vi "Assert ExcelReader Core.vi"() -> ()   [LabVIEW 2015, in "Admin_Actor.lvlib" / "ExcelReader.lvclass"]
uses:
  ExcelReader.lvclass
panel:
  in  "Path":path
  in  "ExcelReader in":refnum<class "ExcelReader.lvclass">
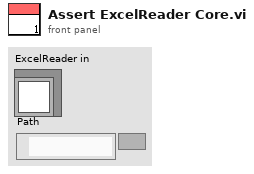
[diagram p1: front panel]
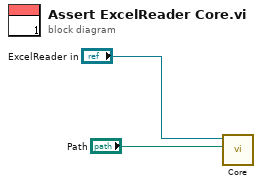
[diagram p0: block diagram]
diagram:
  n1 = call "Core.vi"("Path"="Path", "ExcelReader in"="ExcelReader in") -> ()  [unwired: 7 in, 3 out]
